vi "Invoke Measure Logic.vi"(1 "gRPCid in":T4, 5 "MeasurementPlugin in":refnum<class "MeasurementPluginService.lvclass">, 7 "IMeasurementService in":refnum<class "IMeasurementService.lvclass">, 9 "MeasureRequest":T1, 11 "error in (no error)":errorcluster) -> (6 "Measure Response":T5, 15 "error out":errorcluster)   [LabVIEW 2020, in "MeasurementLink Measurement Server.lvlib" / "IMeasurementService.lvclass"]
uses:
  IMeasurementService.lvclass
  Helpers/TypeDefs/MeasureResponse.ctl
  MeasurementLink Measurement Server Internal/RPC Messages/google_protobuf_Any.ctl
  MeasurementPluginService/MeasurementPluginService.lvclass
  <vilib>/gRPC/LabVIEW gRPC Library/Shared/grpcId.ctl
  Helpers/TypeDefs/MeasureRequest.ctl
  <vilib>/gRPC/LabVIEW gRPC Library/Shared/Any.ctl
  Helpers/TypeDefs/PinMapContext.ctl
  <vilib>/gRPC/LabVIEW gRPC Library/Server API/typeDefs/gRPC Status Code.ctl
  gRPC Utilities/GrpcClientPool/FGV Action.ctl
  MeasurementContext/MeasurementContext.lvclass
  <vilib>/gRPC/LabVIEW gRPC Library/grpc-lvsupport-release.lvlib
  gRPC Utilities/GrpcClientPool/GrpcClientPool.lvclass
  MeasurementLink Measurement Server Internal/MeasurementLink Measurement Server Internal.lvlib
  MeasurementLink Measurement Server.lvlib
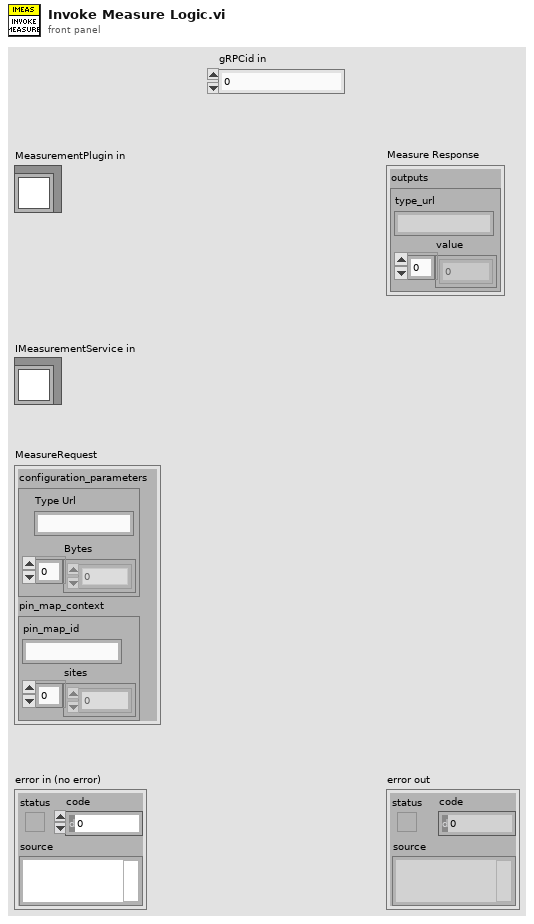
[diagram p1: front panel]
types:
  T1 = typedef "MeasurementLink Measurement Server.lvlib/MeasureRequest.ctl" = cluster{"configuration_parameters":T2, "pin_map_context":T3}
  T2 = typedef "grpc-lvsupport-release.lvlib/Any.ctl" = cluster{"Type Url":string, "Bytes":u8[]}
  T3 = typedef "MeasurementLink Measurement Server.lvlib/PinMapContext.ctl" = cluster{"pin_map_id":string, "sites":i32[]}
  T4 = typedef "grpc-lvsupport-release.lvlib/grpcId.ctl" = u64
  T5 = typedef "MeasurementLink Measurement Server.lvlib/MeasureResponse.ctl" = cluster{"outputs":T6}
  T6 = typedef "MeasurementLink Measurement Server Internal.lvlib/google_protobuf_Any.ctl" = cluster{"type_url":string, "value":u8[]}
  T7 = typedef "gRPC Utilities.lvlib/GrpcClientPool.lvclass/FGV Action.ctl" = enum16{"Get Discovery Client", "Get Session Client", "Get Pinmap Client", "Destroy Clients"}
  T8 = typedef "grpc-lvsupport-release.lvlib/gRPC Status Code.ctl" = enum16{"OK", "CANCELLED", "UNKNOWN", "INVALID_ARGUMENT", "DEADLINE_EXCEEDED", "NOT_FOUND", "ALREADY_EXISTS", "PERMISSION_DENIED", "RESOURCE_EXHAUSTED", "FAILED_PRECONDITION", "ABORTED", "OUT_OF_RANGE", "UNIMPLEMENTED", "INTERNAL", "UNAVAILABLE", "DATA_LOSS", "UNAUTHENTICATED"}
  T9 = typedef "MeasurementLink Measurement Server.lvlib/MeasurementPluginService.lvclass/Plugin Paths.ctl" = cluster{"Get Measurement Details VI Path":path, "Get Type Specializations VI Path":path, "Get UI Details VI Path":path, "Measurement Logic VI Path":path, "Measurement Configuration CTL Path":path, "Measurement Results CTL Path":path}
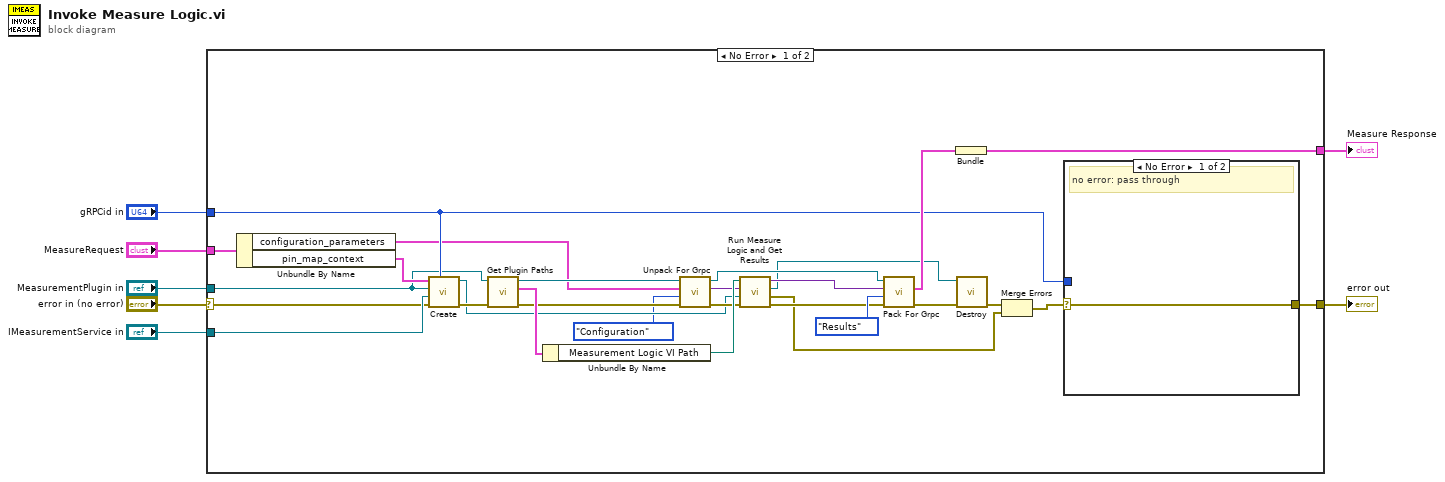
[diagram p0: block diagram]
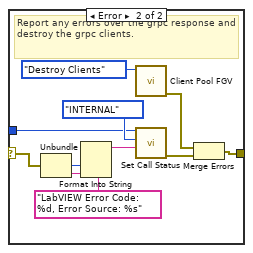
[diagram p2: hidden frame]
diagram:
  n1 = case shown="No Error" "error in (no error)" {
    selector: "error in (no error)" -> [w21 w48]
    tunnel: [w28 w48] -> w6
    tunnel: [w30 _] -> w5
    tunnel: "gRPCid in" -> [w27 _]
    tunnel: "MeasurementPlugin in" -> [w12 _]
    tunnel: "MeasureRequest" -> [w29 _]
    tunnel: "IMeasurementService in" -> [w26 _]
    frame No Error {
      n2 = Unbundle By Name(w29) -> ("configuration_parameters"=w14:T2, "pin_map_context"=w35:T3)
      n3 = call "Create.vi"("gRPC server id"=w27, "error in (no error)"=w21, "IMeasurementService in"=w26, "MeasurementPluginService in"=w12, "pin map context"=w35) -> ("error out"=w34:errorcluster, "MeasurementContext out"=w18:refnum<class "MeasurementContext.lvclass">)  [unwired: 5 in]
      n4 = call-dynamic "Get Plugin Paths.vi"("error in (no error)"=w34, "MeasurementPluginService in"=w12) -> ("error out"=w20:errorcluster, "Plugin Paths"=w31:T9, "MeasurementPluginService out"=w16:refnum<class "MeasurementPluginService.lvclass">)  [unwired: 7 in]
      n5 = Unbundle By Name(w31) -> ("Measurement Logic VI Path"=w24:path)
      n6 = call-dynamic "Unpack For Grpc.vi"("error in (no error)"=w20, "Configuration / Resuls (Config)"=enum16{"Configuration", "Results"}."Configuration", "Any"=w14, "MeasurementPluginService in"=w16) -> ("error out"=w19:errorcluster, "Data Value"=w17:variant, "MeasurementPluginService in"=w15:refnum<class "MeasurementPluginService.lvclass">)  [unwired: 5 in]
      n7 = call "Run Measure Logic and Get Results.vi"("error in (no error)"=w19, "MeasurementContext in"=w18, "Measurement Configuration"=w17, "Measurement Logic VI Path"=w24) -> ("error out"=w23:errorcluster, "Measurement Error"=w8:errorcluster, "MeasurementContext out"=w10:refnum<class "MeasurementContext.lvclass">, "Measurement Output"=w11:variant)  [unwired: 4 in]
      n8 = call-dynamic "Pack For Grpc.vi"("error in (no error)"=w23, "Configuration / Resuls (Config)"=enum16{"Configuration", "Results"}."Results", "Data Value"=w11, "MeasurementPluginService in"=w15) -> ("error out"=w25:errorcluster, "Any"=w33:T2)  [unwired: 5 in, 1 out]
      n9 = Bundle("Any"=w33) -> (w30:cluster{"Any":T2})  [unwired: 1 in]
      n10 = call "Destroy.vi"("error in (no error)"=w25, "MeasurementContext in"=w10) -> ("error out"=w22:errorcluster)  [unwired: 9 in]
      n11 = Merge Errors(w22, w8) -> (w9:errorcluster)
      n12 = case shown="No Error" w9 {
        selector: w9 -> [w36 w41]
        tunnel: [w36 w39] -> w28
        tunnel: w27 -> [_ w40]
        frame No Error {
          # "no error: pass through"
        }
        frame Error {
          # "Report any errors over the grpc response and destroy the grpc clients."
          n13 = Unbundle(w41) -> ("code"=w45:i32, "source"=w46:string)  [unwired: 1 out]
          n14 = Format Into String(format string="LabVIEW Error Code: %d, Error Source: %s", w45, w46) -> (resulting string=w47:string)  [unwired: 2 in, 1 out]
          n15 = call "Client Pool FGV.vi"("Action"=FGV_Action."Destroy Clients") -> ("error out"=w38:errorcluster)  [unwired: 9 in, 1 out]
          n16 = call <vilib>:"Set Call Status.vi"("Details"=w47, "Status Code"=gRPC_Status_Code."INTERNAL", "gRPCid in"=w40) -> ("error out"=w42:errorcluster)  [unwired: 7 in, 1 out]
          n17 = Merge Errors(w38, w42) -> (w39:errorcluster)
        }
      }
    }
    frame Error {
    }
  }
  "error out" <- w6
  "Measure Response" <- w5
